vi "Calc_CMRR.vi"(6 "PGA":i32, 7 "Enable":bool, 8 "error in (no error)":errorcluster, 9 "Input Amplitude(Vpp)":dbl, 10 "Vref (User Entered)":ext, 11 "Fund(dB)":dbl) -> (0 "error out":errorcluster, 2 "CMRR":ext, 3 "PGA Out":i32)   [LabVIEW 2010]
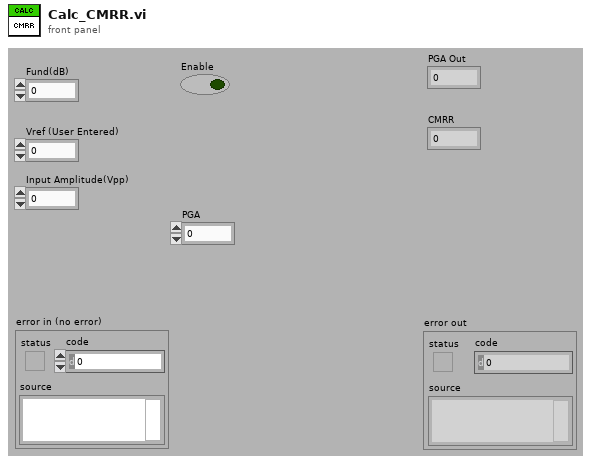
[diagram p1: front panel]
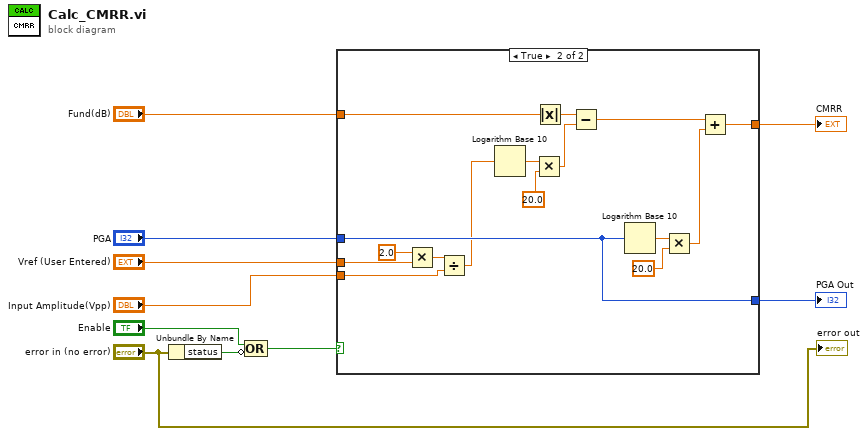
[diagram p0: block diagram]
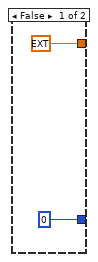
[diagram p2: hidden frame]
diagram:
  n1 = Unbundle By Name("error in (no error)") -> ("status"=w3:bool)
  n2 = Compound Arithmetic op=OR("Enable", invert w3) -> (w4:bool)
  n3 = case shown="True" w4 {
    tunnel: [0 ("PGA") w28] -> w10
    tunnel: [ext 0.0 w27] -> w9
    tunnel: "PGA" -> [_ w28]
    tunnel: "Input Amplitude(Vpp)" -> [_ w26]
    tunnel: "Vref (User Entered)" -> [_ w25]
    tunnel: "Fund(dB)" -> [_ w24]
    frame False {
    }
    frame True {
      n4 = Multiply(x=2.0, y=w25) -> (x*y=w20:ext)
      n5 = Divide(x=w20, y=w26) -> (x/y=w19:ext)
      n6 = Logarithm Base 10(1:w19) -> (0:w23:ext)
      n7 = Multiply(x=w23, y=20.0 ("x")) -> (x*y=w14:ext)
      n8 = Absolute Value(x=w24) -> (abs(x)=w15:dbl)
      n9 = Subtract(x=w15, y=w14) -> (x-y=w13:ext)
      n10 = Logarithm Base 10(1:w28) -> (0:w17:dbl)
      n11 = Multiply(x=w17, y=20.0 ("x")) -> (x*y=w16:dbl)
      n12 = Add(x=w13, y=w16) -> (x+y=w27:ext)
    }
  }
  "PGA Out" <- w10
  "CMRR" <- w9
  "error out" <- "error in (no error)"
